vi "Pre Launch Init.vi"(11 "File Logger in":refnum<class "File Logger.lvclass">) -> (0 "error out":errorcluster, 3 "File Logger out":refnum<class "File Logger.lvclass">)   [LabVIEW 2020, in "Logging.lvlib" / "File Logger.lvclass"]
doc: "(<B>Filename</B>: Actor Framework.lvlib:Actor.lvclass:Pre Launch Init.vi)\n\nDefines behavior that occurs after the Launch Nested Actor method is invoked but before the actor's Actor Core method begins running.\n\nBy default, this method does nothing. A descendant class may override it to define behavior."
uses:
  File Logger.lvclass
  Generic Logger/Generic Logger.lvclass
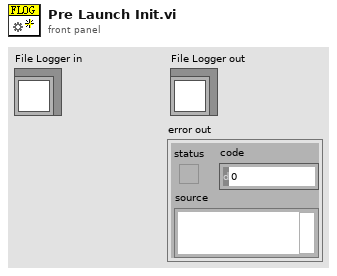
[diagram p1: front panel]
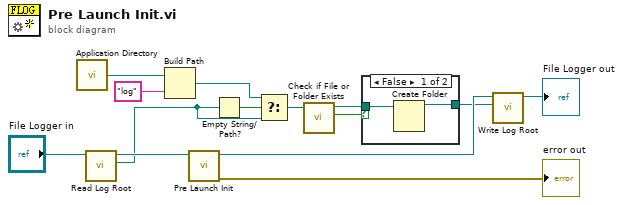
[diagram p0: block diagram]
diagram:
  n1 = call <vilib>:"Application Directory.vi"() -> ("Application Directory"=w13:path)
  n2 = call-dynamic "Read Log Root.vi"("File Logger in"="File Logger in") -> ("Log Root"=w5:path, "File Logger out"=w8:refnum<class "File Logger.lvclass">)  [unwired: 8 in, 1 out]
  n3 = Build Path(base path=w13, name or relative path="log") -> (appended path=w6:path)
  n4 = call-parent "Pre Launch Init.vi"("Logger in"=w8) -> ("error out"=→"error out":errorcluster, "Logger out"=w2:refnum<class "File Logger.lvclass">)  [unwired: 9 in]
  n5 = Empty String/Path?(string/path=w5) -> (empty?=w7:bool)
  n6 = Select(t=w6, s=w7, f=w5) -> (s? t:f=w4:path)
  n7 = call <vilib>:"Check if File or Folder Exists.vi"("path"=w4) -> ("file or folder exists?"=w11:bool, "dup path"=w10:path)  [unwired: 8 in, 1 out]
  n8 = case shown="False" w11 {
    tunnel: w10 -> [w16 w17]
    tunnel: [w15 w17] -> w1
    frame False {
      n9 = Create Folder(path (use dialog)=w16) -> (created path=w15:path)  [unwired: 2 in, 2 out]
    }
    frame True {
    }
  }
  n10 = call-dynamic "Write Log Root.vi"("Log Root"=w1, "File Logger in"=w2) -> ("File Logger out"=→"File Logger out":refnum<class "File Logger.lvclass">)  [unwired: 8 in, 1 out]
